vi "Set FPS.vi"(8 "error in":errorcluster, 11 "IMG_SRC in":refnum<class "IMG_SRC.lvclass">) -> (0 "error out":errorcluster, 2 "Supported?":bool, 3 "IMG_SRC out":refnum<class "IMG_SRC.lvclass">)   [LabVIEW 2018, in "IMG_SRC.lvlib" / "IMG_SRC.lvclass"]
uses:
  IMG_SRC.lvclass
  IMG_SRC.lvclass/IMG_SRC.ctl
  builds/Camera.lvlibp/Camera.lvclass
  C:/Users/Ron.Dexter.LUMINARTECH/Desktop/builds/Camera.lvlibp/Camera.lvclass
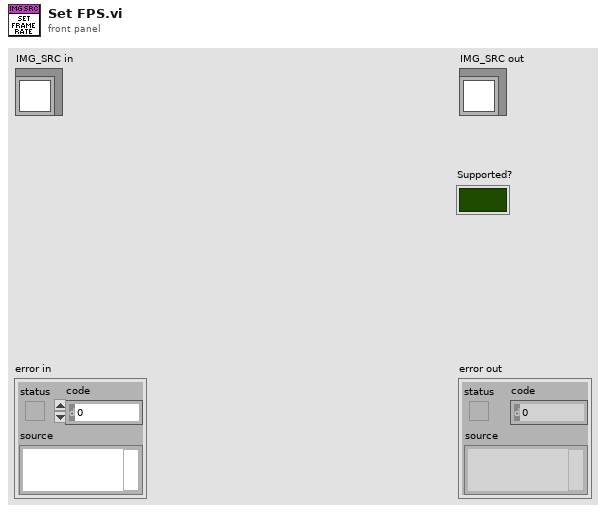
[diagram p1: front panel]
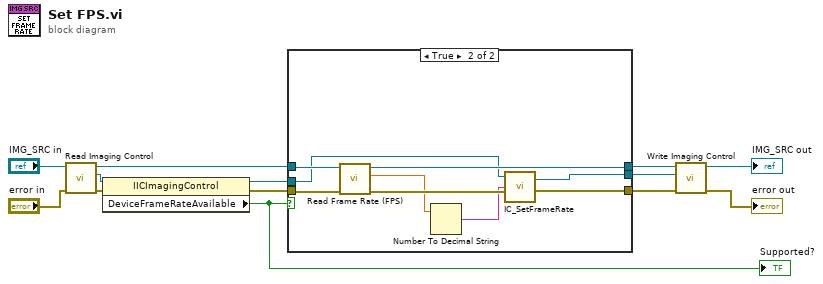
[diagram p0: block diagram]
diagram:
  n1 = call "Read Imaging Control.vi"("error in (no error)"="error in", "IMG_SRC in"="IMG_SRC in") -> ("error out"=w11:errorcluster, "Imaging Control"=w10:refnum<k7>, "IMG_SRC out"=w9:refnum<class "IMG_SRC.lvclass">)  [unwired: 7 in]
  n2 = property class="IICImagingControl"(reference=w10, error in=w11) -> (reference out=w8:refnum<k7>, error out=w7:errorcluster, "DeviceFrameRateAvailable"=w1:bool)
  "Supported?" <- w1
  n3 = case shown="True" w1 {
    tunnel: w9 -> [w14 w22]
    tunnel: w8 -> [w15 w18]
    tunnel: w7 -> [w16 w21]
    tunnel: [w14 w19] -> w4
    tunnel: [w15 w17] -> w3
    tunnel: [w16 w20] -> w2
    frame False {
    }
    frame True {
      n4 = call "Read Frame Rate (FPS).vi"("error in (no error)"=w21, "Camera in"=w22) -> ("error out"=w25:errorcluster, "Frame Rate (FPS)"=w24:dbl, "Camera out"=w19:refnum<class "IMG_SRC.lvclass">)  [unwired: 7 in]
      n5 = Number To Decimal String(number=w24) -> (decimal integer string=w23:string)  [unwired: 1 in]
      n6 = call <userlib>:"IC_SetFrameRate.vi"("Error In (no error)"=w25, "FrameRate"=w23, "ICImagingControl In"=w18) -> ("Error Out"=w20:errorcluster, "ICImagingControl Out"=w17:refnum<k7>)
    }
  }
  n7 = call "Write Imaging Control.vi"("error in (no error)"=w2, "Imaging Control"=w3, "IMG_SRC in"=w4) -> ("error out"=→"error out":errorcluster, "IMG_SRC out"=→"IMG_SRC out":refnum<class "IMG_SRC.lvclass">)  [unwired: 7 in]
